vi "1 Tap 30-Bit RGB.vi"() -> (0 "Pixels":cluster{"Pixel 0":u64})   [LabVIEW 2015]
uses:
  <vilib>/rvi/eio/common/nirviEmuTemplateMethod_errors.vi
  <vilib>/eio/EIONode/EIONode.xnode
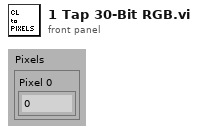
[diagram p1: front panel]
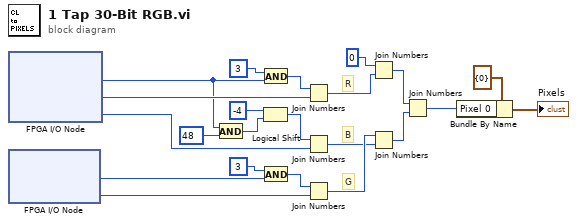
[diagram p0: block diagram]
diagram:
  # "B"
  # "R"
  # "G"
  n1 = xnode "FPGA I/O Node"() -> ("CL Port B"=w7:u8, "CL Port A"=w17:u8, "CL Port C"=w11:u8)  [unwired: 3 in, 3 out]
  n2 = xnode "FPGA I/O Node"() -> ("CL Port F"=w14:u8, "CL Port E"=w13:u8)  [unwired: 2 in, 2 out]
  n3 = And(x=w7, y=u8 48 ("hi")) -> (x .and. y?=w20:u8)
  n4 = Logical Shift(y=i8 -4, x=w20) -> (x << y=w18:u8)
  n5 = And(x=u8 3 ("hi"), y=w7) -> (x .and. y?=w21:u8)
  n6 = And(x=u8 3 ("hi"), y=w14) -> (x .and. y?=w16:u8)
  n7 = Join Numbers(hi=w21, lo=w17) -> ((hi.lo)=w12:u16)
  n8 = Join Numbers(hi=w18, lo=w11) -> ((hi.lo)=w9:u16)
  n9 = Join Numbers(hi=w16, lo=w13) -> ((hi.lo)=w10:u16)
  n10 = Join Numbers(hi=u16 0, lo=w12) -> ((hi.lo)=w5:u32)
  n11 = Join Numbers(hi=w10, lo=w9) -> ((hi.lo)=w4:u32)
  n12 = Join Numbers(hi=w5, lo=w4) -> ((hi.lo)=w3:u64)
  n13 = Bundle By Name(cluster=cluster{"Pixel 0":u64} {"Pixel 0"=0} ("Data"), "Pixel 0"=w3) -> (→"Pixels":cluster{"Pixel 0":u64})
